vi "mod_Narrow Band Low-Pass Filter Design.vi"(0 "Maximum Decimation Factor (512)":enum16{"512", "1024", "2048", "4096"}(ring), 5 "Stop Band Attenuation (120 dB)":T1(ring)=enum."120 dB", 7 "Method (kaiser-sinc)":enum16{"kaiser-sinc", "multi-stage"}(ring), 12 "Alias Protect in Final Transition? (T)":bool=TRUE) -> (4 "Filter Info":cluster{"h":dbl[], "Decimation":dbl} {"h" format="%.2f"; "Decimation" format="%.2f"})   [LabVIEW 2020, in "niAMT.lvlib"]
uses:
  <vilib>/addons/Modulation/niAMT.lvlib
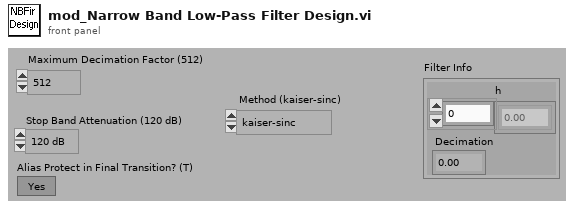
[diagram p1: front panel]
types:
  T1 = enum16{"48 dB", "60 dB", "72 dB", "84 dB", "96 dB", "120 dB"}
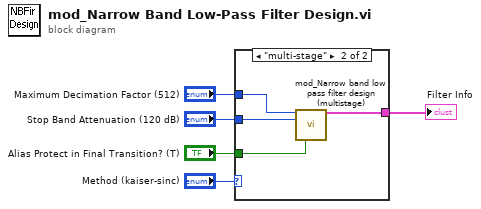
[diagram p0: block diagram]
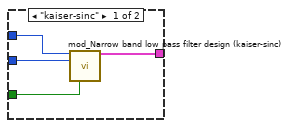
[diagram p2: hidden frame]
diagram:
  n1 = case shown="\"multi-stage\"" "Method (kaiser-sinc)" {
    tunnel: "Maximum Decimation Factor (512)" -> [w9 w12]
    tunnel: "Stop Band Attenuation (120 dB)" -> [w8 w13]
    tunnel: "Alias Protect in Final Transition? (T)" -> [w7 w11]
    tunnel: [w6 w10] -> w1
    frame "kaiser-sinc" {
      n2 = call <vilib>:"mod_Narrow band low pass filter design (kaiser-sinc).vi"("Maximum Decimation Factor (512)"=w9, "Stop Band Attenuation (120 dB)"=w8, "Alias Protect in Final Transition? (T)"=w7) -> ("Filter Info"=w6:cluster{"h":dbl[], "Decimation":dbl})  [unwired: 12 out]
    }
    frame "multi-stage" {
      n3 = call <vilib>:"mod_Narrow band low pass filter design (multistage).vi"("Maximum Decimation Factor (512)"=w12, "Stop Band Attenuation (120 dB)"=w13, "Alias Protect in Final Transition? (T)"=w11) -> ("Filter Info"=w10:cluster{"h":dbl[], "Decimation":dbl})  [unwired: 12 out]
    }
  }
  "Filter Info" <- w1
